vi "Set Test Settings.vi"(10 "Test Settings":T1 {"Lateral Load Cell Sensitivity" format="%.6f"; "Axial Load Cell Sensitivity" format="%.6f"}, 11 "Start Closed Loop Scan Command in":refnum<class "Start Testing Command.lvclass">) -> (3 "Start Closed Loop Scan Command out":refnum<class "Start Testing Command.lvclass">)   [LabVIEW 2015, in "Start Testing Command.lvclass"]
uses:
  Start Testing Command.lvclass
  Typedefs/TestSettings.ctl
  Common_RT_FAILC/DataTypes/FATypes.ctl
  Start Testing Command.lvclass/Start Testing Command.ctl
  Typedefs/FAMT Typedefs.lvlib
  Common_RT_FAILC/RTFAILC.lvlib
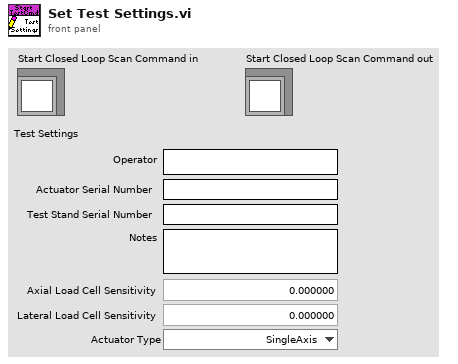
[diagram p1: front panel]
types:
  T1 = typedef "FAMT Typedefs.lvlib/TestSettings.ctl" = cluster{"Operator":string, "Notes":string, "Actuator Serial Number":string, "Test Stand Serial Number":string, "Axial Load Cell Sensitivity":dbl, "Lateral Load Cell Sensitivity":dbl, "Actuator Type":T2}
  T2 = typedef "RTFAILC.lvlib/FATypes.ctl" = enum16{"SingleAxis", "LateralDualAxis", "CrossLateralDualAxis"}
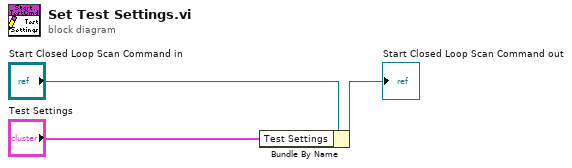
[diagram p0: block diagram]
diagram:
  n1 = Bundle By Name(cluster="Start Closed Loop Scan Command in", "Test Settings"="Test Settings") -> (→"Start Closed Loop Scan Command out":refnum<class "Start Testing Command.lvclass">)
